vi "IRF(X)PSED Guess Parameters v4.vi"(8 "Error In":errorcluster, 9 "X Array":dbl[](array[numeric]), 10 "Y Array":dbl[](array[numeric]), 11 "IRF*PSED fixed Parameters (in)":T1={"order"=0, "T"=0.0, "Time Constant Array"=[], "{S_k, C_k, phi_k, e_k} arrays"={"S_k Array"=[], "C_k Array"=[], "phi_k Array"=[], "e_k Array"=[]}, "IRF Extraction Options"={"Time Constant for IRF Extraction"=1e-18, "IRF Order"=0, "Fourier Series Smoothing"=enum."None", "Noise Threshold"=0.0, "Smoothing Width"=0.0, "Fourier Series Truncation"=enum."Automatic", "Truncation Order"=0, "Save Power Spectrum"=FALSE, "Smoothing"=FALSE, "Smoothing Parameter"=0.0, "Smoothing Order"=1, "Method"=enum."Direct"}} {"IRF Extraction Options"."Smoothing Order" min=1 max=10; "IRF Extraction Options"."Time Constant for IRF Extraction" format="%#_5g"}) -> (0 "Error Out":errorcluster, 2 "Guess Parameters":dbl[](array[numeric]), 3 "IRF*PSED fixed Parameters (out)":T1={"order"=0, "T"=0.0, "Time Constant Array"=[], "{S_k, C_k, phi_k, e_k} arrays"={"S_k Array"=[], "C_k Array"=[], "phi_k Array"=[], "e_k Array"=[]}, "IRF Extraction Options"={"Time Constant for IRF Extraction"=1e-18, "IRF Order"=0, "Fourier Series Smoothing"=enum."None", "Noise Threshold"=0.0, "Smoothing Width"=0.0, "Fourier Series Truncation"=enum."Automatic", "Truncation Order"=0, "Save Power Spectrum"=FALSE, "Smoothing"=FALSE, "Smoothing Parameter"=0.0, "Smoothing Order"=1, "Method"=enum."Direct"}} {"IRF Extraction Options"."Smoothing Order" min=1 max=10; "IRF Extraction Options"."Time Constant for IRF Extraction" format="%#_5g"}, 4 "Parameters Minimum":dbl[](array[numeric]), 6 "Parameters Maximum":dbl[](array[numeric]))   [LabVIEW 2021, in "Fits.lvlib"]
uses:
  IRF(X)PSED Fixed Parameters v3.ctl
  IRF(X)PSED Extraction Options.ctl
  Fourier Series Smoothing Option.ctl
  Fourier Series Truncation.ctl
  IRF Extraction Method.ctl
  Fits.lvlib
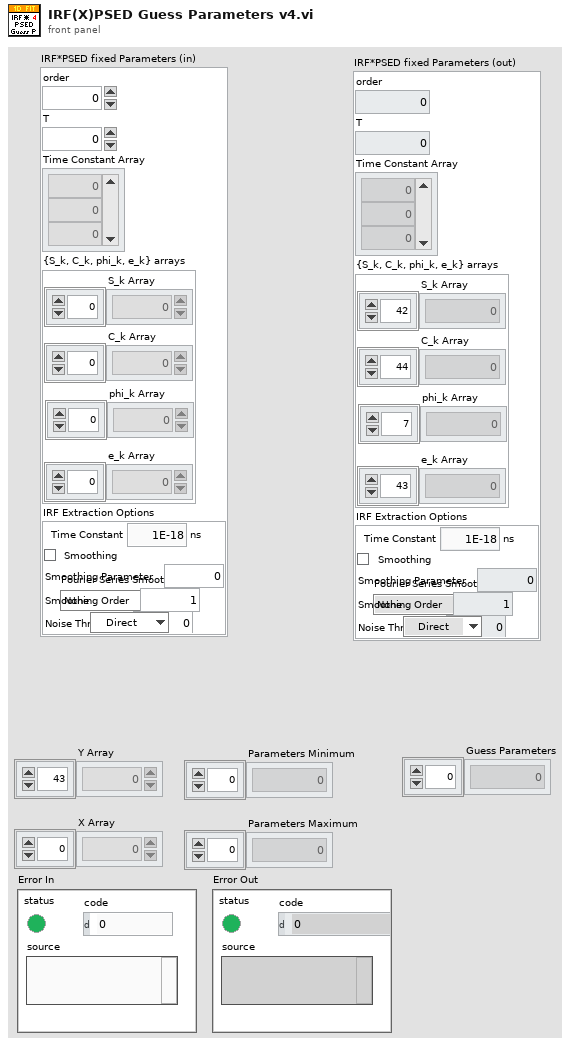
[diagram p1: front panel]
types:
  T1 = typedef "Fits.lvlib/IRF(X)PSED Fixed Parameters v3.ctl" = cluster{"order":i32, "T":dbl, "Time Constant Array":dbl[], "{S_k, C_k, phi_k, e_k} arrays":cluster{"S_k Array":dbl[], "C_k Array":dbl[], "phi_k Array":dbl[], "e_k Array":dbl[]}, "IRF Extraction Options":T2}
  T2 = typedef "Fits.lvlib/IRF(X)PSED Extraction Options.ctl" = cluster{"Time Constant for IRF Extraction":dbl[unit], "IRF Order":i32, "Fourier Series Smoothing":T3, "Noise Threshold":dbl, "Smoothing Width":dbl, "Fourier Series Truncation":T4, "Truncation Order":i32, "Save Power Spectrum":bool, "Smoothing":bool, "Smoothing Parameter":dbl, "Smoothing Order":u32, "Method":T5}
  T3 = typedef "Fits.lvlib/Fourier Series Smoothing Option.ctl" = enum16{"None", "Lanczos Factors", "Fejer Summation"}
  T4 = typedef "Fits.lvlib/Fourier Series Truncation.ctl" = enum16{"Automatic", "Fixed"}
  T5 = typedef "Fits.lvlib/IRF Extraction Method.ctl" = enum16{"Direct", "Topless", "Toeplitz"}
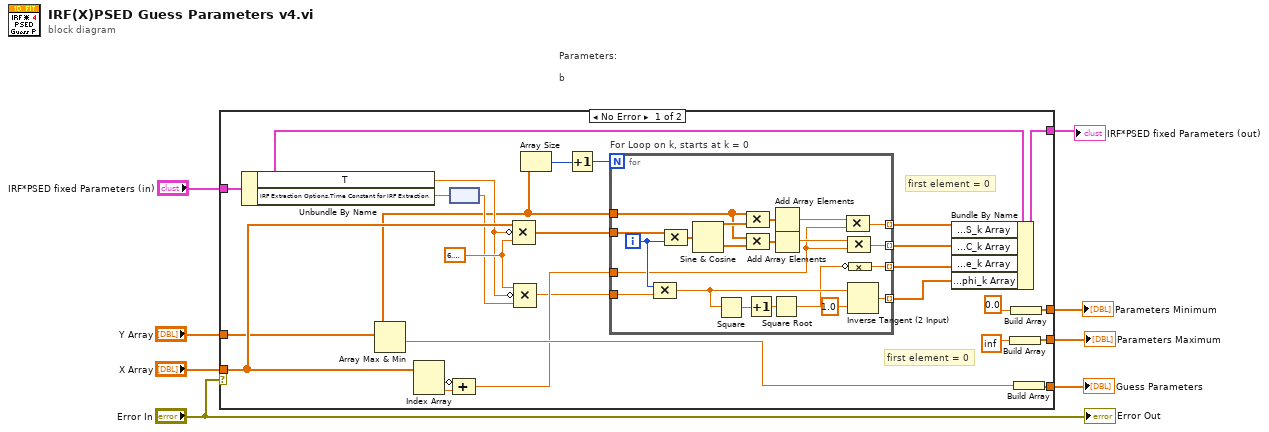
[diagram p0: block diagram]
diagram:
  # "Parameters:\n\nb"
  n1 = case shown="No Error" "Error In" {
    tunnel: [w32 _] -> w8
    tunnel: [w31 _] -> w7
    tunnel: [w30 _] -> w6
    tunnel: "X Array" -> [w25 _]
    tunnel: "Y Array" -> [w11 _]
    tunnel: "IRF*PSED fixed Parameters (in)" -> [w23 w55]
    tunnel: [w24 w55] -> w2
    frame No Error {
      w16 = 6.283185307179586
      # "first element = 0"
      # "first element = 0"
      # "Fixed Parameters:\n\nT, tau, {tau_i}"
      n2 = Unbundle By Name(w23) -> ("T"=w15:dbl, "IRF Extraction Options.Time Constant for IRF Extraction"=w20:dbl[unit])
      n3 = Array Max & Min(array=w11) -> (min value=w29:dbl)  [unwired: 3 out]
      n4 = Index Array(array=w25) -> (element #1=w26:dbl, element #2=w28:dbl)  [unwired: 2 in]
      n5 = node(w20) -> (w12:dbl)
      n6 = Compound Arithmetic op=ADD(invert w26, w28) -> (w22:dbl)
      n7 = Compound Arithmetic op=MULTIPLY(w25, invert w15, w16) -> (w21:dbl[])
      n8 = Compound Arithmetic op=MULTIPLY(w16, invert w15, w12) -> (w19:dbl)
      n9 = Array Size(array=w11) -> (size(s)=w10:i32)
      n10 = Increment(x=w10) -> (x+1=w9:i32)
      n11 = for "For Loop on k, starts at k = 0" {
        N: w9 -> [_]
        tunnel: w21 -> [w54]
        tunnel: w11 -> [w50]
        tunnel: w22 -> [w39]
        tunnel: w19 -> [w47]
        tunnel: [w45] -> w13 mode=indexing
        tunnel: [w38] -> w18 mode=indexing
        tunnel: [w37] -> w17 mode=indexing
        tunnel: [w35] -> w14 mode=indexing
        i -> [w44]
        n12 = Compound Arithmetic op=MULTIPLY(w44, w47) -> (w46:dbl)
        n13 = Compound Arithmetic op=MULTIPLY(w54, w44) -> (w53:dbl[])
        n14 = Sine & Cosine(0:w53) -> (1:w52:dbl[], 2:w51:dbl[])
        n15 = Square(x=w46) -> (x^2=w49:dbl)
        n16 = Increment(x=w49) -> (x+1=w48:dbl)
        n17 = Compound Arithmetic op=MULTIPLY(w50, w52) -> (w43:dbl[])
        n18 = Compound Arithmetic op=MULTIPLY(w50, w51) -> (w42:dbl[])
        n19 = Square Root(x=w48) -> (sqrt(x)=w36:dbl)
        n20 = Add Array Elements(numeric array=w43) -> (sum=w41:dbl)
        n21 = Add Array Elements(numeric array=w42) -> (sum=w40:dbl)
        n22 = Compound Arithmetic op=MULTIPLY(w41, w39) -> (w38:dbl)
        n23 = Compound Arithmetic op=MULTIPLY(w40, w39) -> (w37:dbl)
        n24 = Inverse Tangent (2 Input)(1:1.0 ("x"), 2:w46) -> (0:w45:dbl)
        n25 = Compound Arithmetic op=MULTIPLY(invert w36) -> (w35:dbl)
      }
      n26 = Bundle By Name(cluster=w23, "{S_k, C_k, phi_k, e_k} arrays.S_k Array"=w18, "{S_k, C_k, phi_k, e_k} arrays.C_k Array"=w17, "{S_k, C_k, phi_k, e_k} arrays.e_k Array"=w14, "{S_k, C_k, phi_k, e_k} arrays.phi_k Array"=w13) -> (w24:T1)
      n27 = Build Array(inf ("element")) -> (w32:dbl[])
      n28 = Build Array(0.0 ("element")) -> (w31:dbl[])
      n29 = Build Array(w29) -> (w30:dbl[])
    }
    frame Error {
    }
  }
  "Parameters Maximum" <- w8
  "Parameters Minimum" <- w7
  "Guess Parameters" <- w6
  "IRF*PSED fixed Parameters (out)" <- w2
  "Error Out" <- "Error In"
